vi "Create Helper Loop Events.vi"(11 "Acquisition in":refnum<class "Acquisition.lvclass">) -> (3 "Acquisition out":refnum<class "Acquisition.lvclass">)   [LabVIEW 2018, in "Acquisition.lvlib" / "Acquisition.lvclass"]
uses:
  Acquisition.lvclass
  Acquisition.lvclass/Acquisition.ctl
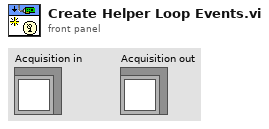
[diagram p1: front panel]
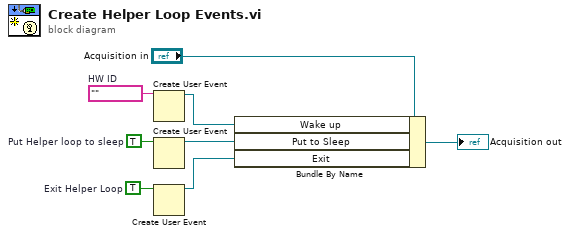
[diagram p0: block diagram]
diagram:
  w7 = TRUE  # Exit Helper Loop
  w3 = TRUE  # Put Helper loop to sleep
  w2 = ""  # HW ID
  n1 = Create User Event(user event datatype=w2) -> (user event=w5:refnum<user-event>)  [unwired: 1 in, 1 out]
  n2 = Create User Event(user event datatype=w3) -> (user event=w6:refnum<user-event>)  [unwired: 1 in, 1 out]
  n3 = Create User Event(user event datatype=w7) -> (user event=w8:refnum<user-event>)  [unwired: 1 in, 1 out]
  n4 = Bundle By Name(cluster="Acquisition in", "Wake up"=w5, "Put to Sleep"=w6, "Exit"=w8) -> (→"Acquisition out":refnum<class "Acquisition.lvclass">)
